vi "Format Setup String.vi"(0 "CS in":refnum<class "CS.lvclass">, 1 "On&G 0":T1, 2 "On&G 1":T1, 3 "On&G 2":T1, 4 "On&G 3":T1, 5 "error in (no error)":errorcluster) -> (14 "CS out":refnum<class "CS.lvclass">, 17 "Setup string":string, 19 "error out":errorcluster)   [LabVIEW 2016, in "CS.lvclass"]
uses:
  Lib.llb/CS.lvclass
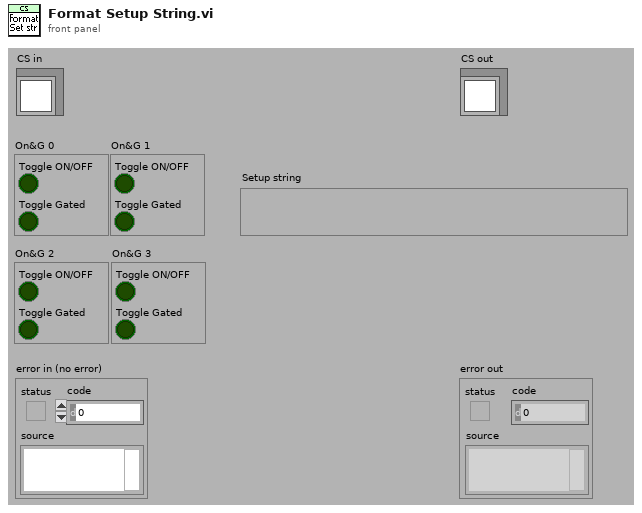
[diagram p1: front panel]
types:
  T1 = cluster{"Toggle ON/OFF":bool, "Toggle Gated":bool}
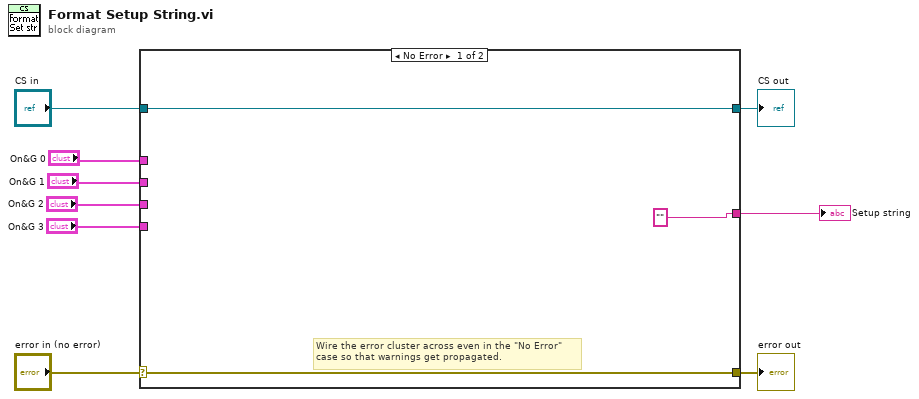
[diagram p0: block diagram]
diagram:
  n1 = case shown="No Error" "error in (no error)" {
    selector: "error in (no error)" -> [w11 w14]
    tunnel: [w11 w14] -> w8
    tunnel: [w12 w13] -> w6
    tunnel: "CS in" -> [w12 w13]
    tunnel: "On&G 0" -> [_ _]
    tunnel: "On&G 1" -> [_ _]
    tunnel: "On&G 2" -> [_ _]
    tunnel: "On&G 3" -> [_ _]
    tunnel: ["" _] -> w1
    frame No Error {
      # "Wire the error cluster across even in the \"No Error\"\ncase so that warnings get propagated."
    }
    frame Error {
    }
  }
  "error out" <- w8
  "CS out" <- w6
  "Setup string" <- w1
